vi "Set Scroll.vi"(8 "error in (no error)":errorcluster, 10 "Position":i32, 11 "ArrayManager in":refnum<class "ArrayManager.lvclass">) -> (0 "error out":errorcluster, 3 "ArrayManager out":refnum<class "ArrayManager.lvclass">)   [LabVIEW 2020, in "OOPanel.lvlib" / "ArrayManager.lvclass"]
uses:
  ArrayManager.lvclass
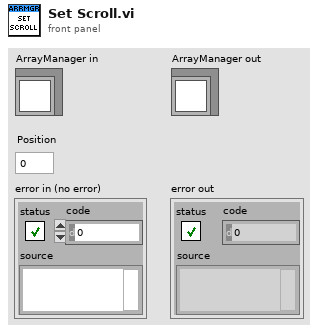
[diagram p1: front panel]
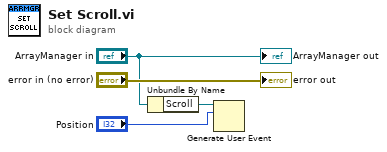
[diagram p0: block diagram]
diagram:
  n1 = Unbundle By Name("ArrayManager in") -> ("Scroll"=w2:refnum<user-event>)
  n2 = Generate User Event(user event=w2, event data cluster="Position") -> ()  [unwired: 2 in, 2 out]
  "error out" <- "error in (no error)"
  "ArrayManager out" <- "ArrayManager in"
